vi "Initialize-object.vi"(6 "Main VI ref":refnum<vi>, 8 "error in (no error)":errorcluster, 9 "Com-in":refnum<queue>, 10 "Com-out":refnum<queue>) -> (0 "error out":errorcluster, 3 "Data ref.":refnum<data-value>)   [LabVIEW 2013, in "CameraVision.lvlib" / "CV-Main.lvclass"]
uses:
  CV-Main.lvclass
  SA-SLMAPI/Sources/Message.lvclass
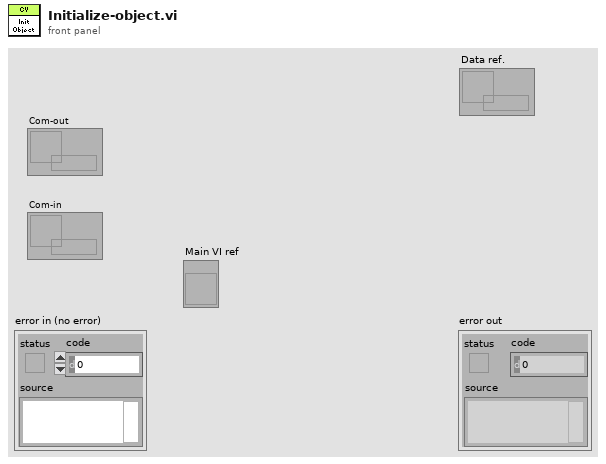
[diagram p1: front panel]
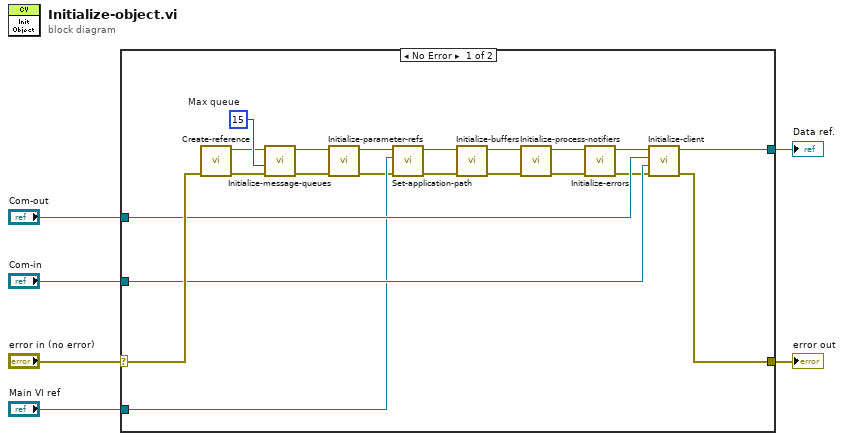
[diagram p0: block diagram]
diagram:
  n1 = case shown="No Error" "error in (no error)" {
    selector: "error in (no error)" -> [w27 w28]
    tunnel: [w20 w28] -> w5
    tunnel: [w21 _] -> w4
    tunnel: "Com-out" -> [w24 _]
    tunnel: "Com-in" -> [w25 _]
    tunnel: "Main VI ref" -> [w17 _]
    frame No Error {
      w26 = 15  # Max queue
      n2 = call "Create-reference.vi"("error in (no error)"=w27) -> ("error out"=w23:errorcluster, "Data ref."=w22:refnum<data-value>)  [unwired: 9 in]
      n3 = call "Initialize-message-queues.vi"("error in"=w23, "Queue depth (15)"=w26, "Data ref. in"=w22) -> ("error IO"=w11:errorcluster, "Data ref."=w12:refnum<data-value>)  [unwired: 6 in, 1 out]
      n4 = call "Initialize-parameter-refs.vi"("error in (no error)"=w11, "Data ref. in"=w12) -> ("error out"=w10:errorcluster, "Data ref."=w9:refnum<data-value>)  [unwired: 8 in]
      n5 = call "Set-application-path.vi"("error in (no error)"=w10, "Main VI ref"=w17, "Data ref. in"=w9) -> ("error out"=w7:errorcluster, "Data ref."=w8:refnum<data-value>)  [unwired: 7 in]
      n6 = call "Initialize-buffers.vi"("error in (no error)"=w7, "Data ref. in"=w8) -> ("error out"=w18:errorcluster, "Data ref."=w19:refnum<data-value>)  [unwired: 8 in]
      n7 = call "Initialize-process-notifiers.vi"("error in (no error)"=w18, "Data ref. in"=w19) -> ("error out"=w14:errorcluster, "Data ref."=w13:refnum<data-value>)  [unwired: 8 in]
      n8 = call "Initialize-errors.vi"("error in (no error)"=w14, "Data ref. in"=w13) -> ("error out"=w15:errorcluster, "Data ref."=w16:refnum<data-value>)  [unwired: 8 in]
      n9 = call "Initialize-client.vi"("error in (no error)"=w15, "Client channel"=w25, "Server channel"=w24, "Data ref. in"=w16) -> ("error out"=w20:errorcluster, "Data ref."=w21:refnum<data-value>)  [unwired: 6 in]
    }
    frame Error {
    }
  }
  "error out" <- w5
  "Data ref." <- w4
